vi "AgB29xx_LabVIEW_SinusoidalWaveform.vi"() -> ()   [LabVIEW 2009]
panel:
  out "Measurement Voltage":bool=TRUE
  out "Sinusoidal Waveform Data (Volts)":dbl[](array[numeric])
  in  "Timer (sec)":dbl=0.01
  in  "Measurement Trigger Source":i32(ring)=19 items=["AgB29xxArmTriggerSourceInt1"=0, "AgB29xxArmTriggerSourceInt2"=1, "AgB29xxArmTriggerSourceExt1"=2, "AgB29xxArmTriggerSourceExt2"=3, "AgB29xxArmTriggerSourceExt3"=4, "AgB29xxArmTriggerSourceExt4"=5, "AgB29xxArmTriggerSourceExt5"=6, "AgB29xxArmTriggerSourceExt6"=7, "AgB29xxArmTriggerSourceExt7"=8, "AgB29xxArmTriggerSourceExt8"=9, "AgB29xxArmTriggerSourceExt9"=10, "AgB29xxArmTriggerSourceExt10"=11, "AgB29xxArmTriggerSourceExt11"=12, "AgB29xxArmTriggerSourceExt12"=13, "AgB29xxArmTriggerSourceExt13"=14, "AgB29xxArmTriggerSourceExt14"=15, "AgB29xxArmTriggerSourceAint"=17, "AgB29xxArmTriggerSourceBus"=18, "AgB29xxArmTriggerSourceTimer"=19]
  in  "Measurement Trigger Count":i32=100
  in  "Transient Trigger Source":i32(ring)=17 items=["AgB29xxArmTriggerSourceInt1"=0, "AgB29xxArmTriggerSourceInt2"=1, "AgB29xxArmTriggerSourceExt1"=2, "AgB29xxArmTriggerSourceExt2"=3, "AgB29xxArmTriggerSourceExt3"=4, "AgB29xxArmTriggerSourceExt4"=5, "AgB29xxArmTriggerSourceExt5"=6, "AgB29xxArmTriggerSourceExt6"=7, "AgB29xxArmTriggerSourceExt7"=8, "AgB29xxArmTriggerSourceExt8"=9, "AgB29xxArmTriggerSourceExt9"=10, "AgB29xxArmTriggerSourceExt10"=11, "AgB29xxArmTriggerSourceExt11"=12, "AgB29xxArmTriggerSourceExt12"=13, "AgB29xxArmTriggerSourceExt13"=14, "AgB29xxArmTriggerSourceExt14"=15, "AgB29xxArmTriggerSourceAint"=17, "AgB29xxArmTriggerSourceBus"=18, "AgB29xxArmTriggerSourceTimer"=19]
  in  "Transient Trigger Count":i32=1
  in  "Compliance Value (Amps)":dbl=0.1
  in  "NPLC Current":dbl=0.1
  in  "Frequency (Hz)":dbl=1.0
  in  "Amplitude (V)":dbl=1.0
  out "NumberOfChannels":i32
  in  "OptionString":string=" DriverSetup= Model=, Trace=false"
  in  "Simulate":bool=TRUE
  in  "AgB29xxLib.IAgB29xx2":refnum<k7>
  out "Simulate":bool=TRUE
  out "Vendor":string="Agilent Technologies"
  in  "IdQuery":bool=TRUE
  in  "Reset":bool=TRUE
  in  "ResourceName":string="GPIB0::23::INSTR"
  out "SerialNumber":string="0123456789"
  out "Identifier":string="AgM9216"
  out "InstrumentFirmwareRevision":string="Sim1.0.5.0"
  out "InstrumentModel":string="M9216A"
  out "Revision":string="1.0.5.0"
  out "Description":string="IVI Driver for Agilent M9216"
  # "SinusoidalWaveform"
  # "Configure Sinusoidal Waveform"
  # "Configure Voltage Measurement"
  # "Configure Trigger"
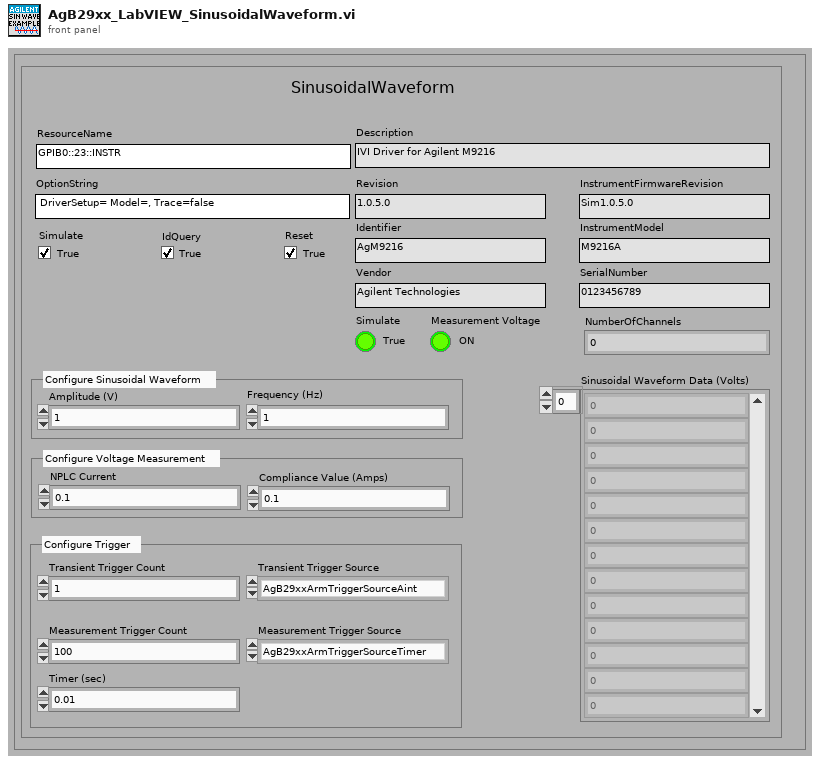
[diagram p1: front panel]
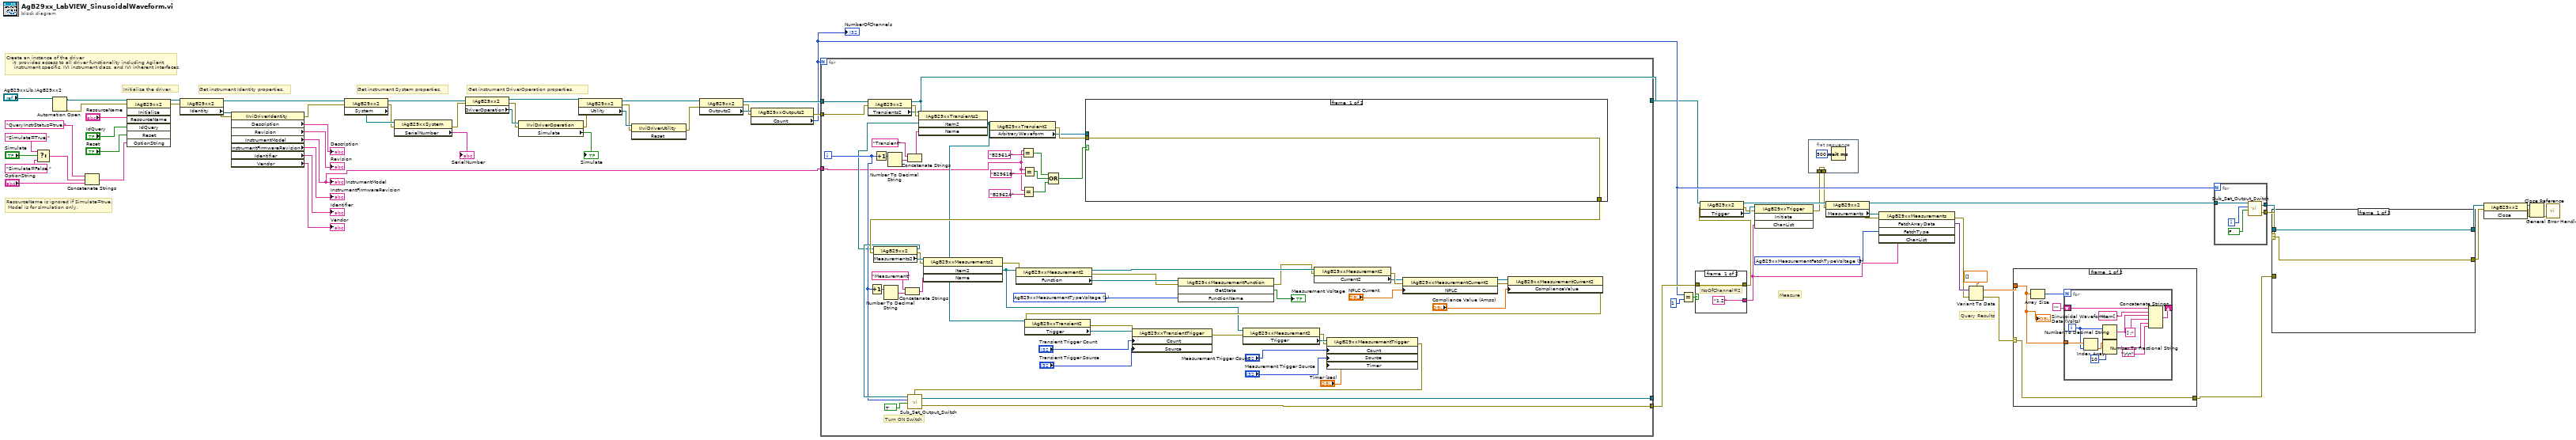
[diagram p0: block diagram]
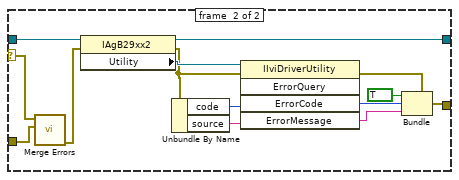
[diagram p2: hidden frame]
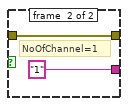
[diagram p4: hidden frame]
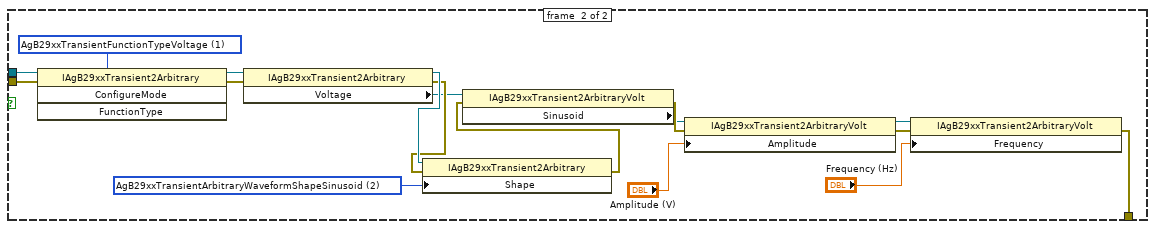
[diagram p5: hidden frame]
diagram:
  w25 = 5 items=["AgB29xxMeasurementFetchTypeCurrent", "AgB29xxMeasurementFetchTypeResistance", "AgB29xxMeasurementFetchTypeSource", "AgB29xxMeasurementFetchTypeStatus", "AgB29xxMeasurementFetchTypeTime", "AgB29xxMeasurementFetchTypeVoltage", "AgB29xxMeasurementFetchTypeAll"] ("FetchType")
  # "Query Results"
  # "Measure"
  # "Get instrument DriverOperation properties."
  # "ResourceName is ignored if Simulate=true.\n Model is for simulation only."
  # "Get instrument System properties."
  # "Get instrument Identity properties."
  # "Initialize the driver."
  # "Create an instance of the driver\n    it  provides access to all driver functionality including Agilent\n     instrument specific, IVI instrument class, and IVI inherent interfaces."
  n1 = Select(t="Simulate=True,", s="Simulate", f="Simulate=False,") -> (s? t:f=w42:string)
  n2 = Automation Open(Automation Refnum="AgB29xxLib.IAgB29xx2") -> (Automation Refnum=w49:refnum<k7>, error out=w48:errorcluster)  [unwired: 3 in]
  n3 = Concatenate Strings("QueryInstrStatus=true," ("string"), w42, "OptionString") -> (w40:string)
  n4 = invoke class="IAgB29xx2" method="Initialize"(reference=w49, error in=w48, "ResourceName"="ResourceName", "IdQuery"="IdQuery", "Reset"="Reset", "OptionString"=w40) -> (reference out=w66:refnum<k7>, error out=w62:errorcluster)  [unwired: 1 in, 5 out]
  n5 = property class="IAgB29xx2"(reference=w66, error in=w62) -> (reference out=w58:refnum<k7>, error out=w59:errorcluster, "Identity"=w69:refnum<k7>)
  n6 = property class="IIviDriverIdentity"(reference=w69, error in=w59) -> (error out=w52:errorcluster, "Description"=→"Description":string, "Revision"=→"Revision":string, "InstrumentModel"=w1:string, "InstrumentFirmwareRevision"=→"InstrumentFirmwareRevision":string, "Identifier"=→"Identifier":string, "Vendor"=→"Vendor":string)  [unwired: 1 out]
  "InstrumentModel" <- w1
  n7 = property class="IAgB29xx2"(reference=w58, error in=w52) -> (reference out=w56:refnum<k7>, error out=w51:errorcluster, "System"=w57:refnum<k7>)
  n8 = property class="IAgB29xxSystem"(reference=w57, error in=w51) -> (error out=w54:errorcluster, "SerialNumber"=→"SerialNumber":string)  [unwired: 1 out]
  n9 = property class="IAgB29xx2"(reference=w56, error in=w54) -> (reference out=w47:refnum<k7>, error out=w53:errorcluster, "DriverOperation"=w55:refnum<k7>)
  n10 = property class="IIviDriverOperation"(reference=w55, error in=w53) -> (error out=w46:errorcluster, "Simulate"=→"Simulate":bool)  [unwired: 1 out]
  n11 = property class="IAgB29xx2"(reference=w47, error in=w46) -> (reference out=w36:refnum<k7>, error out=w37:errorcluster, "Utility"=w38:refnum<k7>)
  n12 = invoke class="IIviDriverUtility" method="Reset"(reference=w38, error in=w37) -> (error out=w34:errorcluster)  [unwired: 1 in, 2 out]
  n13 = property class="IAgB29xx2"(reference=w36, error in=w34) -> (reference out=w32:refnum<k7>, error out=w33:errorcluster, "Outputs2"=w35:refnum<k7>)
  n14 = property class="IAgB29xxOutputs2"(reference=w35, error in=w33) -> (error out=w31:errorcluster, "Count"=w8:i32)  [unwired: 1 out]
  "NumberOfChannels" <- w8
  n15 = for {
    N: w8 -> [_]
    tunnel: w32 -> [w94]
    tunnel: w31 -> [w126]
    tunnel: [w89] -> w9
    tunnel: [w90] -> _
    tunnel: [w81] -> w4
    tunnel: w1 -> [w73]
    i -> [w88]
    w83 = u16 1 items=["AgB29xxMeasurementTypeVoltage"=1] ("Configure FunctionType")
    # "Turn ON Switch"
    n16 = property class="IAgB29xx2"(reference=w94, error in=w126) -> (reference out=w81:refnum<k7>, error out=w128:errorcluster, "Transients2"=w127:refnum<k7>)
    n17 = Increment(x=w88) -> (x+1=w119:i32)
    n18 = Increment(x=w88) -> (x+1=w125:i32)
    n19 = Number To Decimal String(number=w119) -> (decimal integer string=w118:string)  [unwired: 1 in]
    n20 = Number To Decimal String(number=w125) -> (decimal integer string=w124:string)  [unwired: 1 in]
    n21 = Concatenate Strings("Measurement" ("string"), w118) -> (w87:string)
    n22 = Concatenate Strings("Transient" ("string"), w124) -> (w122:string)
    n23 = invoke class="IAgB29xxTransients2" method="Item2"(reference=w127, error in=w128, "Name"=w122) -> ("Item2"=w107:refnum<k7>)  [unwired: 1 in, 3 out]
    n24 = property class="IAgB29xxTransient2"(reference=w107) -> (error out=w130:errorcluster, "ArbitraryWaveform"=w129:refnum<k7>)  [unwired: 1 in, 1 out]
    n25 = Equal?(x=w73, y="B2961A" ("string")) -> (x = y?=w78:bool)
    n26 = Equal?(x=w73, y="B2962A" ("string")) -> (x = y?=w80:bool)
    n27 = Equal?(x=w73, y="B2961B" ("string")) -> (x = y?=w79:bool)
    n28 = Compound Arithmetic op=OR(w78, w79, w80) -> (w74:bool)
    n29 = case shown="True" w74 {
      tunnel: w130 -> [w131 w143]
      tunnel: w129 -> [_ w142]
      tunnel: [w131 w132] -> w112
      frame #0 {
      }
      frame #1 {
        w135 = 2 items=["AgB29xxTransientArbitraryWaveformShapeExponent", "AgB29xxTransientArbitraryWaveformShapeRamp", "AgB29xxTransientArbitraryWaveformShapeSinusoid", "AgB29xxTransientArbitraryWaveformShapeSquare", "AgB29xxTransientArbitraryWaveformShapeTrapezoid", "AgB29xxTransientArbitraryWaveformShapeTriangle", "AgB29xxTransientArbitraryWaveformShapeUserDefined"] ("WaveformShape")
        w145 = 1 items=["AgB29xxTransientFunctionTypeCurrent", "AgB29xxTransientFunctionTypeVoltage"] ("Configure FunctionType")
        n30 = invoke class="IAgB29xxTransient2Arbitrary" method="ConfigureMode"(reference=w142, error in=w143, "FunctionType"=w145) -> (reference out=w138:refnum<k7>, error out=w144:errorcluster)  [unwired: 1 in, 2 out]
        n31 = property class="IAgB29xxTransient2Arbitrary"(reference=w138, error in=w144) -> (reference out=w137:refnum<k7>, error out=w136:errorcluster, "Voltage"=w133:refnum<k7>)
        n32 = property class="IAgB29xxTransient2Arbitrary"(reference=w137, error in=w136, "Shape"=w135) -> (error out=w134:errorcluster)  [unwired: 1 out]
        n33 = property class="IAgB29xxTransient2ArbitraryVolt"(reference=w133, error in=w134) -> (error out=w140:errorcluster, "Sinusoid"=w139:refnum<k7>)  [unwired: 1 out]
        n34 = property class="IAgB29xxTransient2ArbitraryVolt"(reference=w139, error in=w140, "Amplitude"="Amplitude (V)") -> (reference out=w146:refnum<k7>, error out=w147:errorcluster)
        n35 = property class="IAgB29xxTransient2ArbitraryVolt"(reference=w146, error in=w147, "Frequency"="Frequency (Hz)") -> (error out=w132:errorcluster)  [unwired: 1 out]
      }
    }
    n36 = property class="IAgB29xx2"(reference=w81, error in=w112) -> (reference out=w93:refnum<k7>, error out=w120:errorcluster, "Measurements2"=w121:refnum<k7>)
    n37 = invoke class="IAgB29xxMeasurements2" method="Item2"(reference=w121, error in=w120, "Name"=w87) -> (error out=w116:errorcluster, "Item2"=w101:refnum<k7>)  [unwired: 1 in, 2 out]
    n38 = property class="IAgB29xxMeasurement2"(reference=w101, error in=w116) -> (reference out=w115:refnum<k7>, error out=w84:errorcluster, "Function"=w85:refnum<k7>)
    n39 = invoke class="IAgB29xxMeasurementFunction" method="GetState"(reference=w85, error in=w84, "FunctionName"=w83) -> (error out=w86:errorcluster, "GetState"=→"Measurement Voltage":bool)  [unwired: 1 in, 2 out]
    n40 = property class="IAgB29xxMeasurement2"(reference=w115, error in=w86) -> (error out=w114:errorcluster, "Current2"=w113:refnum<k7>)  [unwired: 1 out]
    n41 = property class="IAgB29xxMeasurementCurrent2"(reference=w113, error in=w114, "NPLC"="NPLC Current") -> (reference out=w110:refnum<k7>, error out=w109:errorcluster)
    n42 = property class="IAgB29xxMeasurementCurrent2"(reference=w110, error in=w109, "ComplianceValue"="Compliance Value (Amps)") -> (error out=w106:errorcluster)  [unwired: 1 out]
    n43 = property class="IAgB29xxTransient2"(reference=w107, error in=w106) -> (error out=w105:errorcluster, "Trigger"=w104:refnum<k7>)  [unwired: 1 out]
    n44 = property class="IAgB29xxTransientTrigger"(reference=w104, error in=w105, "Count"="Transient Trigger Count", "Source"="Transient Trigger Source") -> (error out=w100:errorcluster)  [unwired: 1 out]
    n45 = property class="IAgB29xxMeasurement2"(reference=w101, error in=w100) -> (error out=w95:errorcluster, "Trigger"=w99:refnum<k7>)  [unwired: 1 out]
    n46 = property class="IAgB29xxMeasurementTrigger"(reference=w99, error in=w95, "Count"="Measurement Trigger Count", "Source"="Measurement Trigger Source", "Timer"="Timer (sec)") -> (error out=w91:errorcluster)  [unwired: 1 out]
    n47 = call "Sub_Set_Output_Switch.vi"("error in"=w91, "Enabled? (False)"=TRUE ("Enabled"), "i"=w88, "AgB29xxLib.IAgB29xx2"=w93) -> ("error out"=w89:errorcluster, "AgB29xxLib.IAgB29xx2 2"=w90:refnum<k7>)
  }
  n48 = Equal?(x=w8, y=1 ("iStart")) -> (x = y?=w18:bool)
  n49 = case shown="False" w18 {
    tunnel: ["1,2" "1"] -> w15
    tunnel: w9 -> [w149 w151]
    tunnel: [w149 w151] -> w16
    frame #0 {
      # "NoOfChannel=2"
    }
    frame #1 {
      # "NoOfChannel=1"
    }
  }
  n50 = property class="IAgB29xx2"(reference=w4, error in=w16) -> (reference out=w26:refnum<k7>, error out=w22:errorcluster, "Trigger"=w28:refnum<k7>)
  n51 = invoke class="IAgB29xxTrigger" method="Initiate"(reference=w28, error in=w22, "ChanList"=w15) -> (error out=w7:errorcluster)  [unwired: 1 in, 3 out]
  n52 = flat-sequence {
    tunnel: w7 -> [w153]
    tunnel: [w153] -> w6
    frame #0 {
      n53 = Wait (ms)(milliseconds to wait=u32 500) -> ()  [unwired: 1 out]
    }
  }
  n54 = property class="IAgB29xx2"(reference=w26, error in=w6) -> (reference out=w5:refnum<k7>, error out=w21:errorcluster, "Measurements"=w27:refnum<k7>)
  n55 = invoke class="IAgB29xxMeasurements" method="FetchArrayData"(reference=w27, error in=w21, "FetchType"=w25, "ChanList"=w15) -> (error out=w19:errorcluster, "FetchArrayData"=w23:variant)  [unwired: 1 in, 3 out]
  n56 = Variant To Data(error in=w19, Variant=w23, type=dbl[] []) -> (error out=w2:errorcluster, data=w14:dbl[])
  n57 = case shown="No Error" w2 {
    selector: w2 -> [w157 w170]
    tunnel: w14 -> [w156 _]
    tunnel: [w157 w170] -> w3
    frame #0 {
      n58 = Array Size(array=w156) -> (size(s)=w155:i32)
      n59 = for {
        N: w155 -> [_]
        tunnel: w156 -> [w165]
        shift-right: [w162] -> _
        shift-left: "" -> [w161]
        i -> [w160]
        n60 = Index Array(array=w165, index=w160) -> (element=w164:dbl)
        n61 = Number To Decimal String(number=w160) -> (decimal integer string=w168:string)  [unwired: 1 in]
        n62 = Number To Fractional String(number=w164, precision (6)=i16 10) -> (F-format string=w166:string)  [unwired: 2 in]
        n63 = Concatenate Strings(w161, "Item[ " ("string"), w168, "] :" ("string"), w166, "\r\n") -> (w162:string)
      }
      "Sinusoidal Waveform Data (Volts)" <- w156
    }
    frame #1 {
    }
  }
  n64 = for {
    N: w8 -> [_]
    tunnel: w5 -> [w175]
    tunnel: [w173] -> w13
    tunnel: [w172] -> w12
    i -> [w171]
    n65 = call "Sub_Set_Output_Switch.vi"("Enabled? (False)"=FALSE ("AutoRangeEnabled"), "i"=w171, "AgB29xxLib.IAgB29xx2"=w175) -> ("error out"=w173:errorcluster, "AgB29xxLib.IAgB29xx2 2"=w172:refnum<k7>)  [unwired: 1 in]
  }
  n66 = case shown="Error" w13 {
    selector: w13 -> [w176 w179]
    tunnel: [w176 w181] -> w10
    tunnel: w12 -> [w177 w191]
    tunnel: [w177 w189] -> w11
    tunnel: w3 -> [_ w180]
    frame #0 {
    }
    frame #1 {
      n67 = call <vilib>:"Merge Errors.vi"("error in 2 (no error)"=w180, "error in 1 (no error)"=w179) -> ("error out"=w178:errorcluster)  [unwired: 5 in]
      n68 = property class="IAgB29xx2"(reference=w191, error in=w178) -> (reference out=w189:refnum<k7>, error out=w186:errorcluster, "Utility"=w190:refnum<k7>)
      n69 = Unbundle By Name(w186) -> ("code"=w188:i32, "source"=w187:string)
      n70 = invoke class="IIviDriverUtility" method="ErrorQuery"(reference=w190, error in=w186, "ErrorCode"=w188, "ErrorMessage"=w187) -> (error out=w182:errorcluster, "ErrorCode"=w185:i32, "ErrorMessage"=w184:string)  [unwired: 1 in, 2 out]
      n71 = Bundle(cluster=w182, "status"=TRUE, "code"=w185, "source"=w184) -> (w181:errorcluster)
    }
  }
  n72 = invoke class="IAgB29xx2" method="Close"(reference=w11, error in=w10) -> (reference out=w30:refnum<k7>, error out=w29:errorcluster)  [unwired: 1 in, 1 out]
  n73 = Close Reference(reference=w30, error in (no error)=w29) -> (error out=w20:errorcluster)
  n74 = call <vilib>:"General Error Handler.vi"("error in (no error)"=w20) -> ()  [unwired: 10 in, 5 out]
